vi "Read.vi"(8 "error in (no error)":errorcluster, 11 "Bronkhorst Settings in":T1={"VISA resource name"="", "Simulated?"=FALSE, "Smoothing Steps"=1} {"Smoothing Steps" min=1 step=1}) -> (0 "error out":errorcluster, 1 "Connection Error":bool, 2 "flow":dbl, 3 "Bronkhorst Settings out":T1={"VISA resource name"="", "Simulated?"=FALSE, "Smoothing Steps"=1} {"Smoothing Steps" min=1 step=1})   [LabVIEW 2018, in "Bronkhorst M13 Flow Meter.lvlib"]
uses:
  Bronkhorst M13 Flow Meter.lvlib
  Settings Cluster.ctl
  <userlib>/_OpenG.lib/numeric/numeric.llb/Random Number Within Range - DBL__ogtk.vi
  <vilib>/regexp/Match Regular Expression.xnode
  <vilib>/ptbypt/NI_PtbyPt.lvlib
panel:
  out "x/y":dbl
  out "whole match":string
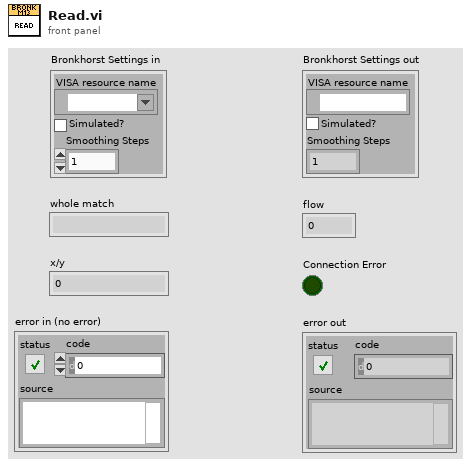
[diagram p1: front panel]
types:
  T1 = typedef "Bronkhorst M13 Flow Meter.lvlib/Settings Cluster.ctl" = cluster{"VISA resource name":refnum<visa-resource-name>, "Simulated?":bool, "Smoothing Steps":i32}
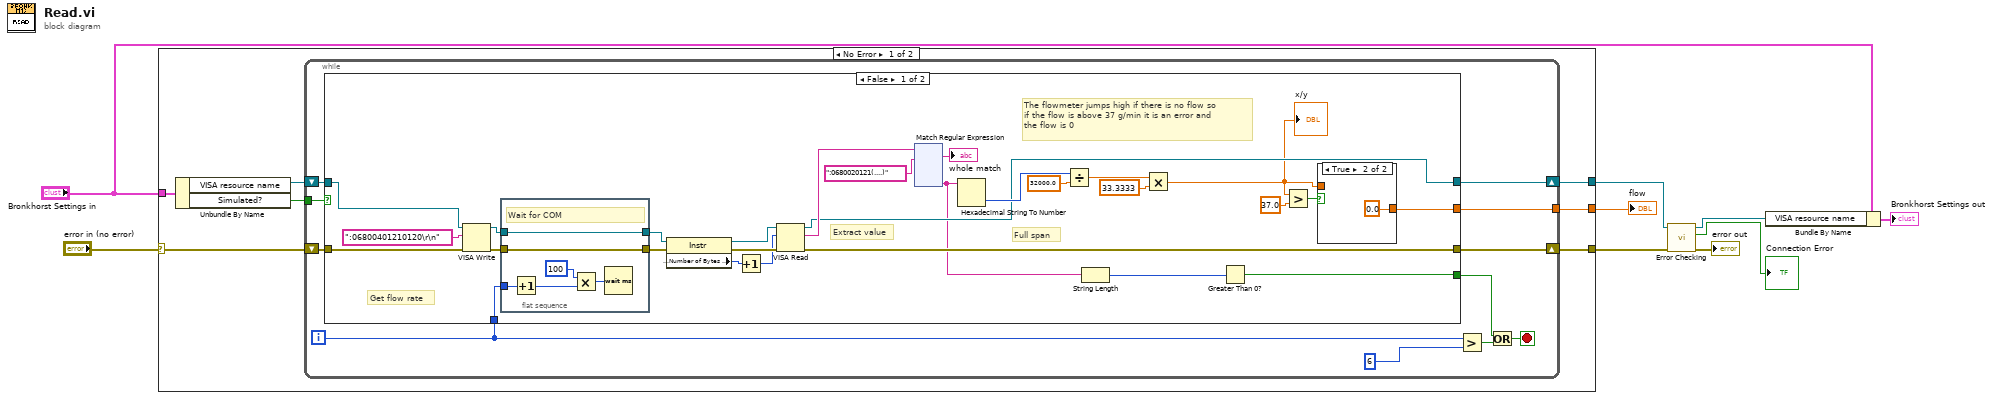
[diagram p0: block diagram]
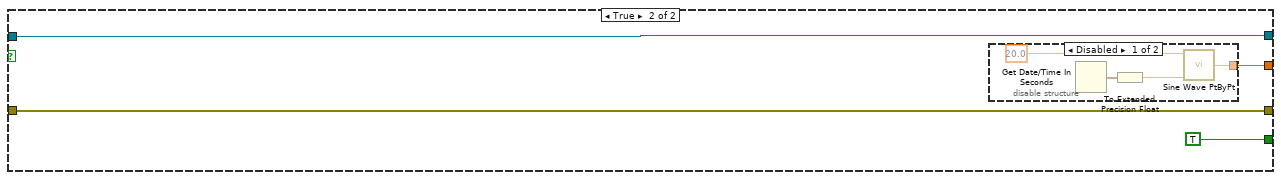
[diagram p3: hidden frame]
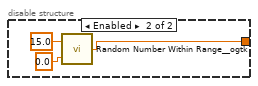
[diagram p4: hidden frame]
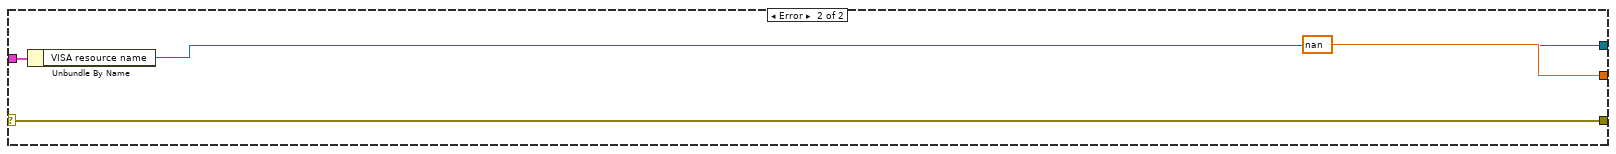
[diagram p5: hidden frame]
diagram:
  n1 = case shown="No Error" "error in (no error)" {
    selector: "error in (no error)" -> [w15 w194]
    tunnel: [w14 w194] -> w3
    tunnel: "Bronkhorst Settings in" -> [w12 w192]
    tunnel: [w13 nan ("sine wave")] -> w9
    tunnel: [w10 w191] -> w5
    frame No Error {
      n2 = Unbundle By Name(w12) -> ("VISA resource name"=w11:refnum<visa-resource-name>, "Simulated?"=w16:bool)
      n3 = while {
        tunnel: w16 -> [w27]
        tunnel: [w24] -> w13
        shift-right: [w25] -> w14
        shift-left: w15 -> [w26]
        shift-right: [w22] -> w10
        shift-left: w11 -> [w23]
        i -> [w18]
        stop <- w17 stop-if-true
        n4 = case shown="False" w27 {
          tunnel: [w33 w183] -> w25
          tunnel: w26 -> [w38 w183]
          tunnel: [w42 w182] -> w24
          tunnel: [w34 w181] -> w22
          tunnel: w23 -> [w39 w181]
          tunnel: [w28 TRUE] -> w19
          tunnel: w18 -> [w30 _]
          frame False {
            # "Full span"
            # "Extract value"
            # "Get flow rate"
            # "The flowmeter jumps high if there is no flow so \nif the flow is above 37 g/min it is an error and \nthe flow is 0"
            n5 = VISA Write(VISA resource name=w39, write buffer=":06800401210120\r\n" ("Command"), error in (no error)=w38) -> (VISA resource name out=w52:refnum<visa-resource-name>, error out=w50:errorcluster)  [unwired: 1 out]
            n6 = flat-sequence {
              tunnel: [w179] -> w51
              tunnel: w52 -> [w179]
              tunnel: [w178] -> w49
              tunnel: w50 -> [w178]
              tunnel: w30 -> [w175]
              frame #0 {
                # "Wait for COM"
                n7 = Increment(x=w175) -> (x+1=w174:i32)
                n8 = Multiply(x=u32 100 ("milliseconds to wait"), y=w174) -> (x*y=w176:u32)
                n9 = Wait (ms)(milliseconds to wait=w176) -> ()  [unwired: 1 out]
              }
            }
            n10 = property class="Instr"(reference=w51, error in=w49) -> (reference out=w54:refnum<visa-resource-name>, error out=w53:errorcluster, "Serial Settings:Number of Bytes at Serial Port"=w36:u32)
            n11 = Increment(x=w36) -> (x+1=w35:u32)
            n12 = VISA Read(VISA resource name=w54, byte count=w35, error in (no error)=w53) -> (VISA resource name out=w34:refnum<visa-resource-name>, read buffer=w37:string, error out=w33:errorcluster)  [unwired: 1 out]
            n13 = xnode "Match Regular Expression"("input string"=w37, "regular expression"=":0680020121(....)" ("Regular Expression for Extracting Weight")) -> ("whole match"=→"whole match":string, "submatch 1"=w31:string)  [unwired: 4 in, 4 out]
            n14 = Hexadecimal String To Number(string=w31) -> (number=w40:u32)  [unwired: 2 in, 1 out]
            n15 = Divide(x=w40, y=32000.0) -> (x/y=w44:dbl)
            n16 = String Length(string=w31) -> (length=w29:i32)
            n17 = Multiply(x=w44, y=33.3333) -> (x*y=w32:dbl)
            "x/y" <- w32
            n18 = Greater Than 0?(x=w29) -> (x > 0?=w28:bool)
            n19 = Greater?(x=w32, y=37.0) -> (0:w43:bool)
            n20 = case shown="True" w43 {
              tunnel: [w56 0.0] -> w42
              tunnel: w32 -> [w56 _]
              frame False {
              }
              frame True {
              }
            }
          }
          frame True {
            n21 = disable-structure shown="Disabled" {
              disable-tunnel: [w184 w188] -> w182
              frame Disabled {
                n22 = Get Date/Time In Seconds() -> (seconds since 1Jan1904=w187:timestamp)
                n23 = To Extended Precision Float(1:w187) -> (0:w186:ext)
                n24 = call <vilib>:"Sine Wave PtByPt.vi"("time"=w186, "amplitude"=20.0) -> ("sine wave"=w184:dbl)  [unwired: 2 in]
              }
              frame Enabled {
                n25 = call-poly <userlib>:"Random Number Within Range__ogtk.vi"("High"=15.0, "Low"=0.0) -> ("Random Number"=w188:dbl)  [unwired: 3 in]
              }
            }
          }
        }
        n26 = Greater?(x=w18, y=6) -> (0:w20:bool)
        n27 = Or(x=w19, y=w20) -> (x .or. y?=w17:bool)
      }
    }
    frame Error {
      n28 = Unbundle By Name(w192) -> ("VISA resource name"=w191:refnum<visa-resource-name>)
    }
  }
  "flow" <- w9
  n29 = call "Error Checking.vi"("error in (no error)"=w3, "VISA resource name"=w5) -> ("error out"=→"error out":errorcluster, "Connection Error"=→"Connection Error":bool, "VISA resource name"=w4:refnum<visa-resource-name>)  [unwired: 7 in]
  n30 = Bundle By Name(cluster="Bronkhorst Settings in", "VISA resource name"=w4) -> (→"Bronkhorst Settings out":T1)
